vi "TestPublishRate.vi"(8 "error in (no error)":errorcluster, 11 "TestPublishRate In":refnum<class "TestPublishRate.lvclass">) -> (0 "error out":errorcluster, 3 "TestPublishRate Out":refnum<class "TestPublishRate.lvclass">)   [LabVIEW 2015, in "TestPublishRate.lvclass"]
uses:
  TestPublishRate.lvclass
  Framework/IViewModel/IViewModel/IViewModel.lvclass
  Framework/IViewable/IViewable/IViewable.lvclass
  Doubles/TestModelFastPublish/TestModelFastPublish.lvclass
  Framework/Mediator/Mediator/Mediator.lvclass
  Framework/SubscriptionPolicy/ValueChangeSubscription/ValueChangeSubscription.lvclass/ValueChangeSubscription.ctl
  Framework/IViewModel/IViewModel/IViewModel.lvclass/IViewModel.ctl
  Framework/IViewManager/IViewManager Messages/Launch Nested Views Msg/Launch Nested Views Msg.lvclass/Launch Nested Views Msg.ctl
  Framework/IViewManager/IViewManager/IViewManager.lvclass/IViewManager.ctl
  Framework/IObserver/IObserver Messages/Subscribe Msg/Subscribe Msg.lvclass/Subscribe Msg.ctl
  <vilib>/ActorFramework/Message Enqueuer/Message Enqueuer.lvclass/Message Enqueuer.ctl
  <vilib>/ActorFramework/Stop Msg/Stop Msg.lvclass/Stop Msg.ctl
  <vilib>/Analysis/baseanly.llb/Mean (DBL).vi
  Framework/IViewManager/IViewManager Messages/Launch Nested Views Msg/Pack Launch Nested Views Msg.vi
  Framework/IViewManager/IViewManager/Write Startup Launch Nested Views Msg.vi
  <vilib>/ActorFramework/Message Enqueuer/Enqueue.vi
  <vilib>/ActorFramework/Message Enqueuer/Enqueue Critical.vi
  <vilib>/ActorFramework/Message Priority Queue/Priority Enqueue.vi
  Framework/IViewManager/IViewManager Messages/Launch Nested Views Msg/Launch Nested Views Msg.lvclass
  Framework/SubscriptionPolicy/ValueChangeSubscription/ValueChangeSubscription.lvclass
  Framework/IObserver/IObserver Messages/Subscribe Msg/Subscribe Msg.lvclass
  <vilib>/ActorFramework/Stop Msg/Stop Msg.lvclass
  Framework/Transport/QueueTransport/QueueTransport.lvclass
  <vilib>/ActorFramework/Actor/Actor.lvclass
  Framework/IMediator/SubscriptionRequest/SubscriptionRequest.lvclass
  Framework/IMediator/ISubscriptionPolicy/ISubscriptionPolicy.lvclass
  <vilib>/Analysis/NI_AALBase.lvlib
panel:
  out "Iteration":i32
  out "Transmission Times":dbl[](graph)
  out "Actual Publish Period":dbl[](graph)
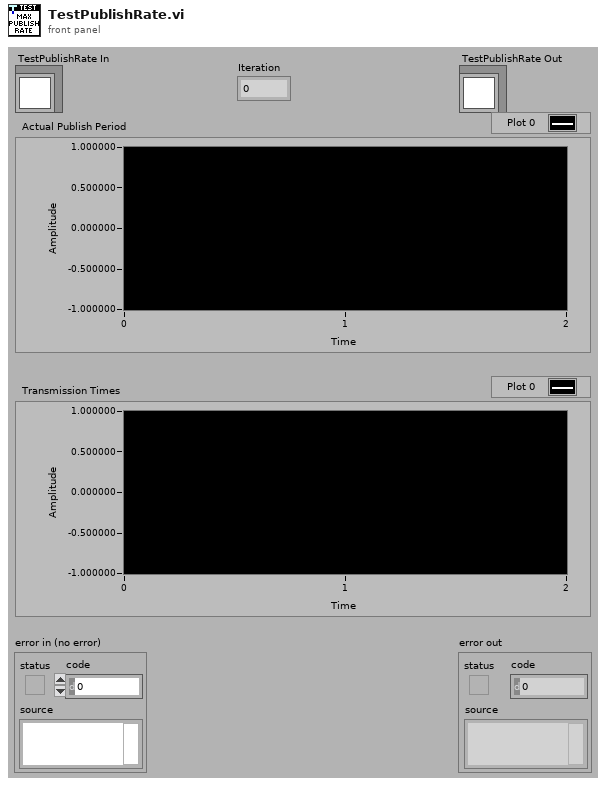
[diagram p1: front panel]
types:
  T1 = typedef "IMediator.lvlib/ISubscriptionPolicy.lvclass/ISubscriptionPolicy Reference.ctl" = refnum<data-value>
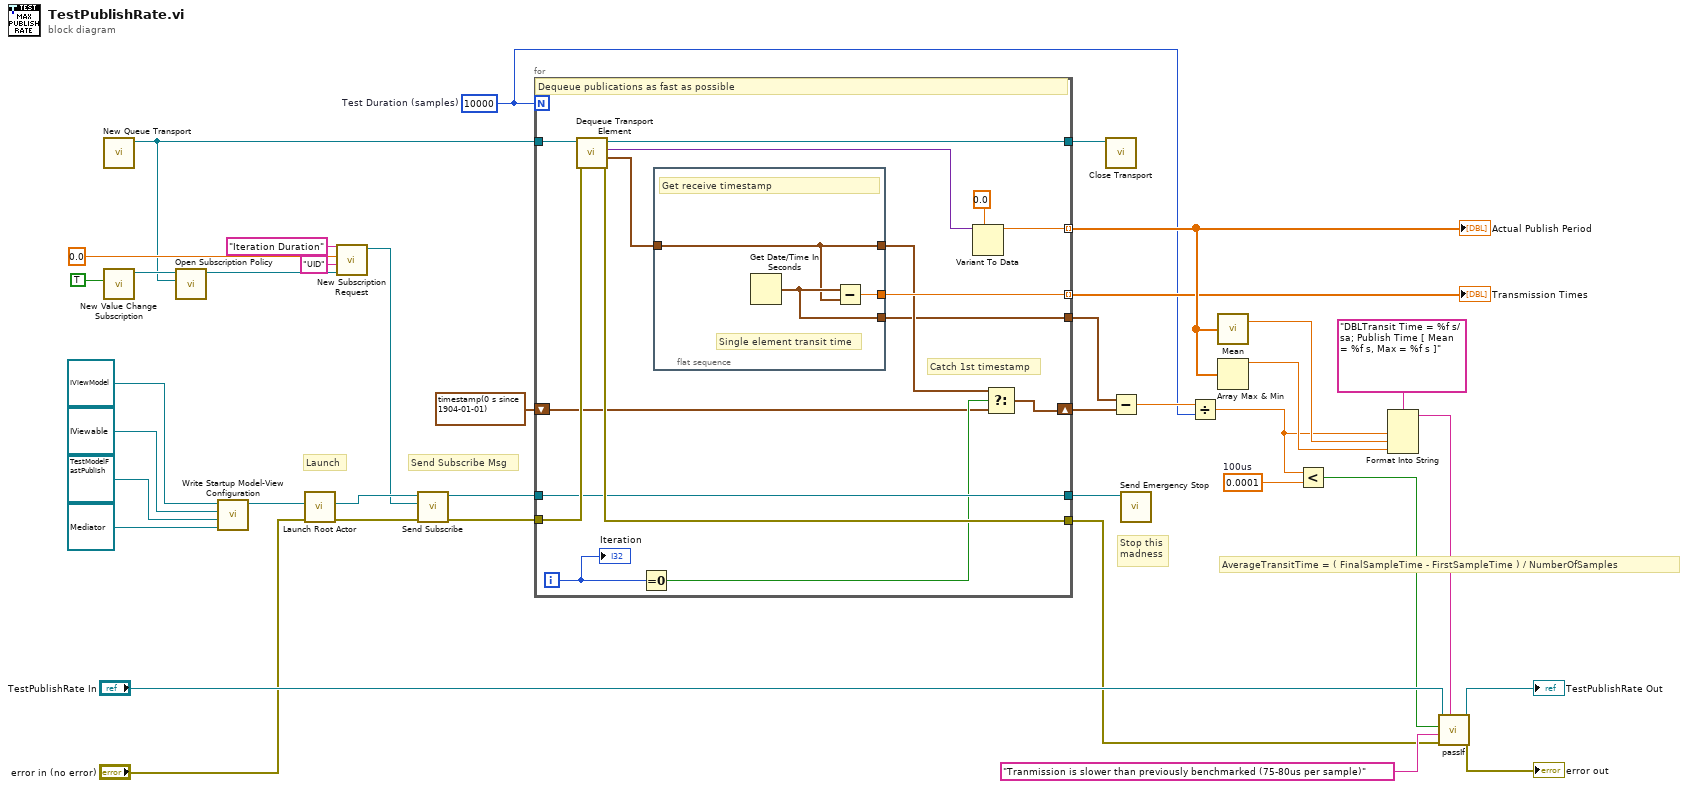
[diagram p0: block diagram]
diagram:
  w7 = 0.0001  # 100us
  w3 = 10000  # Test Duration (samples)
  # "AverageTransitTime = ( FinalSampleTime - FirstSampleTime ) / NumberOfSamples"
  # "Stop this\nmadness"
  # "Send Subscribe Msg"
  # "Launch"
  n1 = call "New Queue Transport.vi"() -> ("QueueTransport Out"=w2:refnum<class "QueueTransport.lvclass">)  [unwired: 10 in, 1 out]
  n2 = call "New Value Change Subscription.vi"("Ignore Past Updates? (F)"=TRUE) -> ("ValueChangeSubscription Out"=w30:refnum<class "ValueChangeSubscription.lvclass">)  [unwired: 10 in]
  n3 = call "Open Subscription Policy.vi"("Transport"=w2, "SubscriptionPolicy"=w30) -> ("Subscription Policy"=w29:T1)  [unwired: 8 in, 1 out]
  n4 = call "Write Startup Model-View Configuration.vi"("Mediator Type"=refnum<class "Mediator.lvclass"> refnum ("Mediator"), "Model Type"=refnum<class "TestModelFastPublish.lvclass"> refnum ("Model"), "Startup View Configuration"=refnum<class "IViewable.lvclass"> refnum, "IViewModel In"=refnum<class "IViewModel.lvclass"> refnum) -> ("IViewModel Out"=w32:refnum<class "IViewModel.lvclass">)  [unwired: 7 in]
  n5 = call <vilib>:"Launch Root Actor.vi"("error in (no error)"="error in (no error)", "Actor"=w32) -> ("error out"=w24:errorcluster, "Actor's Enqueuer"=w31:refnum<class "Message Enqueuer.lvclass">)  [unwired: 8 in]
  n6 = call "New Subscription Request.vi"("Subscription Policy"=w29, "Subscriber ID"="UID" ("Unique Subscriber ID"), "Type"=0.0, "Datum Name"="Iteration Duration" ("Topic Name")) -> ("SubscriptionRequest"=w26:refnum<class "SubscriptionRequest.lvclass">)  [unwired: 7 in]
  n7 = call "Send Subscribe.vi"("error in (no error)"=w24, "SubscriptionRequest"=w26, "Message Enqueuer"=w31) -> ("error out"=w23:errorcluster, "Message Enqueuer out"=w25:refnum<class "Message Enqueuer.lvclass">)  [unwired: 7 in]
  n8 = for {
    N: w3 -> [_]
    tunnel: w25 -> [w50]
    tunnel: w23 -> [w54]
    tunnel: w2 -> [w55]
    tunnel: [w52] -> w17 mode=indexing
    tunnel: [w51] -> w14 mode=indexing
    tunnel: [w53] -> w4
    tunnel: [w50] -> w16
    tunnel: [w49] -> w15
    shift-right: [w48] -> w11
    shift-left: timestamp(0 s since 1904-01-01) ("Publication Time") -> [w44]
    tunnel: [w43] -> w12
    i -> [w46]
    # "Catch 1st timestamp"
    # "Dequeue publications as fast as possible"
    n9 = call "Dequeue Transport Element.vi"("error in (no error)"=w54, "QueueTransport in"=w55) -> ("error out"=w53:errorcluster, "Publication Time"=w41:timestamp, "Data"=w40:variant, "QueueTransport out"=w49:refnum<class "QueueTransport.lvclass">)  [unwired: 6 in]
    n10 = Equal To 0?(x=w46) -> (x = 0?=w45:bool)
    n11 = flat-sequence {
      tunnel: [w58] -> w51
      tunnel: [w56] -> w47
      tunnel: [w57] -> w43
      tunnel: w41 -> [w56]
      frame #0 {
        # "Single element transit time"
        # "Get receive timestamp"
        n12 = Get Date/Time In Seconds() -> (seconds since 1Jan1904=w57:timestamp)
        n13 = Subtract(x=w57, y=w56) -> (x-y=w58:dbl)
      }
    }
    n14 = Variant To Data(type=0.0, Variant=w40) -> (data=w52:dbl)  [unwired: 1 in, 1 out]
    n15 = Select(t=w47, s=w45, f=w44) -> (s? t:f=w48:timestamp)
    "Iteration" <- w46
  }
  "Actual Publish Period" <- w17
  "Transmission Times" <- w14
  n16 = call-dynamic "Close Transport.vi"("QueueTransport in"=w15) -> ()  [unwired: 10 in, 1 out]
  n17 = Subtract(x=w12, y=w11) -> (x-y=w10:dbl)
  n18 = call <vilib>:"Send Emergency Stop.vi"("Message Enqueuer"=w16) -> ()  [unwired: 10 in, 1 out]
  n19 = Divide(x=w10, y=w3) -> (x/y=w8:dbl)
  n20 = call-poly <vilib>:"Mean.vi"("X"=w17) -> ("mean"=w19:dbl)  [unwired: 1 out]
  n21 = Array Max & Min(array=w17) -> (max value=w18:dbl)  [unwired: 3 out]
  n22 = Less?(x=w8, y=w7) -> (x < y?=w6:bool)
  n23 = Format Into String(format string="DBLTransit Time = %f s/sa; Publish Time [ Mean = %f s, Max = %f s ]", w8, w19, w18) -> (resulting string=w9:string)  [unwired: 2 in, 1 out]
  n24 = call-dynamic "passIf.vi"("custom report message (\"\")"=w9, "error in (no error)"=w4, "message (\"\")"="Tranmission is slower than previously benchmarked (75-80us per sample)" ("message (\"\")"), "pass"=w6, "TestCase in"="TestPublishRate In") -> ("error out"=→"error out":errorcluster, "TestCase out"=→"TestPublishRate Out":refnum<class "TestPublishRate.lvclass">)  [unwired: 5 in]
